vi "Variant to Samples Event.vi"(8 "error in (no error)":errorcluster, 10 "Variant":variant, 11 "Samples in":refnum<class "Samples.lvclass">) -> (0 "error out":errorcluster, 2 "Event Registration Refnum":refnum<event-registration>, 3 "Samples out":refnum<class "Samples.lvclass">)   [LabVIEW 2015, in "AMS UI.lvlib" / "Samples.lvclass"]
uses:
  Samples.lvclass
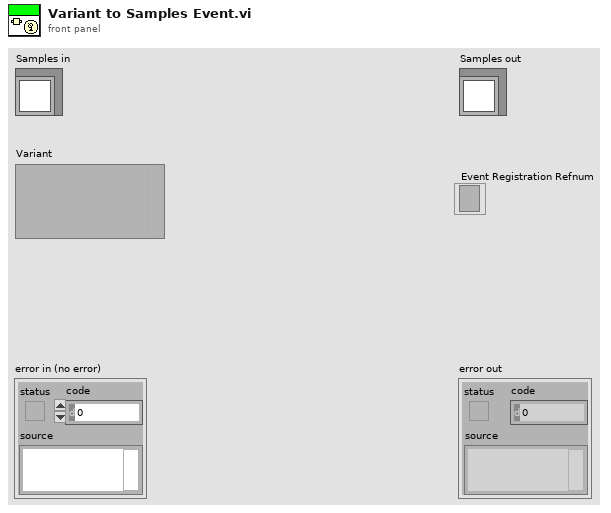
[diagram p1: front panel]
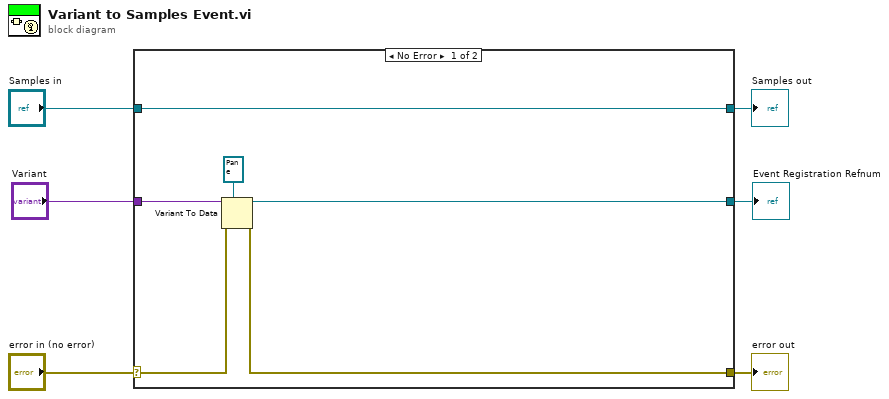
[diagram p0: block diagram]
diagram:
  n1 = case shown="No Error" "error in (no error)" {
    selector: "error in (no error)" -> [w10 w14]
    tunnel: [w9 w14] -> w5
    tunnel: [w12 w13] -> w3
    tunnel: "Samples in" -> [w12 w13]
    tunnel: "Variant" -> [w11 _]
    tunnel: [w8 _] -> w1
    frame No Error {
      n2 = Variant To Data(error in=w10, type=refnum<event-registration> refnum ("event registration refnum"), Variant=w11) -> (data=w8:refnum<event-registration>, error out=w9:errorcluster)
    }
    frame Error {
    }
  }
  "error out" <- w5
  "Samples out" <- w3
  "Event Registration Refnum" <- w1
